vi "Pulse Configure Trigger.vi"(8 "error in":errorcluster, 10 "RFSG session in":refnum<k15>, 11 "RFmx session in":refnum<k21>) -> (0 "error out":errorcluster, 2 "RFSG session out":refnum<k15>, 3 "RFmx session out":refnum<k21>)   [LabVIEW 2023]
uses:
  <instrlib>/niRFSG/niRFSG.llb/niRFSG Signal Names.ctl
  <instrlib>/niRFSG/niRFSG.llb/niRFSG Signal Identifiers.ctl
  <vilib>/RFmx/Pulse/mx/RFmxPulse.llb/RFmxPulse Configure Digital Edge Trigger.vi
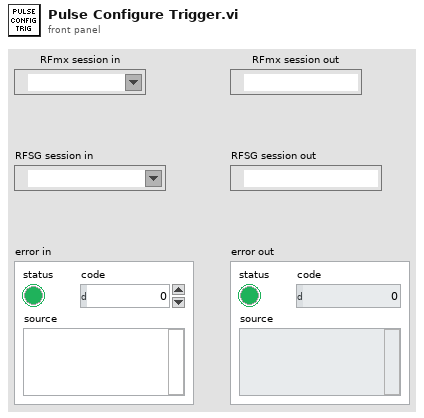
[diagram p1: front panel]
types:
  T1 = typedef "niRFSG Signal Identifiers.ctl" = string
  T2 = typedef "niRFSG Signal Names.ctl" = i32
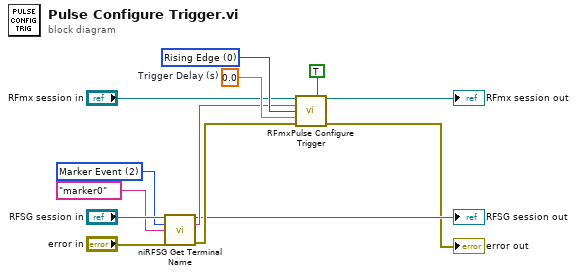
[diagram p0: block diagram]
diagram:
  w6 = T2 2 items=["Start Trigger", "Script Trigger", "Marker Event", "Ref Clock", "Started Event", "Done Event", "Configuration List Step Trigger", "Configuration Settled Event"] ("signal")
  w11 = 0.0  # Trigger Delay (s)
  w12 = 0 items=["Rising Edge", "Falling Edge"] ("Digital Edge")
  n1 = call <instrlib>:"niRFSG Get Terminal Name.vi"("instrument handle"="RFSG session in", "signal"=w6, "signal identifier"=T1 "marker0", "error in"="error in") -> ("instrument handle out"=→"RFSG session out":refnum<k15>, "terminal name"=w7:string, "error out"=w4:errorcluster)  [unwired: 9 in]
  n2 = call-poly <vilib>:"RFmxPulse Configure Trigger.vi"("Instrument Handle In"="RFmx session in", "Enable Trigger?"=TRUE ("IQ Power Edge Enable"), "Digital Edge Source"=w7, "Digital Edge"=w12, "Trigger Delay (s)"=w11, "error in (no error)"=w4) -> ("Instrument Handle Out"=→"RFmx session out":refnum<k21>, "error out"=→"error out":errorcluster)  [unwired: 8 in]
